vi "asset.update.vi"(8 "error in":errorcluster, 11 "Client in":refnum<class "Client.lvclass">) -> (0 "error out":errorcluster, 3 "Client out":refnum<class "Client.lvclass">)   [LabVIEW 2020, in "Client.lvclass"]
doc: "Updates an asset's name and/or description and returns a handle to the updated asset."
uses:
  Client.lvclass
  client.lvlib
panel:
  out "out_asset out":i32
  in  "rid":string
  in  "name":string
  in  "description":string
  in  "out_asset":i32
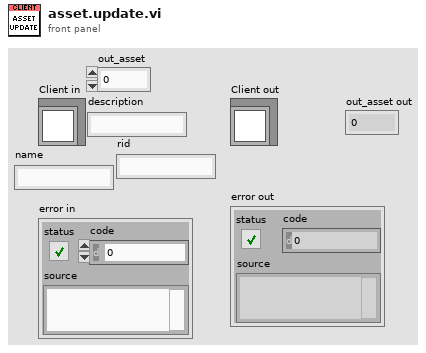
[diagram p1: front panel]
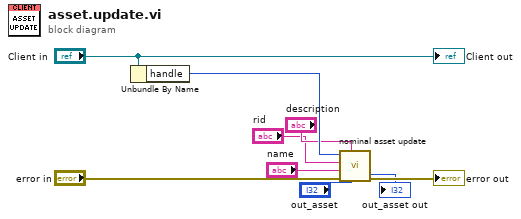
[diagram p0: block diagram]
diagram:
  n1 = Unbundle By Name("Client in") -> ("handle"=w7:i32)
  n2 = call "nominal asset update.vi"("out_asset"="out_asset", "description"="description", "error in (no error)"="error in", "name"="name", "rid"="rid", "client"=w7) -> ("error out"=→"error out":errorcluster, "out_asset out"=→"out_asset out":i32)  [unwired: 3 in, 1 out]
  "Client out" <- "Client in"
